vi "GLdrv_TRIG_COND_CH.vi"(0 "Connection ID":T2, 5 "COND":i32=1 min=0 max=1, 7 "CH":i32=1 min=1, 9 "Set":T1, 11 "error in (no error)":errorcluster, 13 "Query(f)":bool) -> (4 "Connection ID Out":T2, 10 "Set out":T1, 15 "error out":errorcluster)   [LabVIEW 2017, in "GL860_Driver.lvlib"]
doc: "トリガ SourceがAMPに設定されている場合、各アナログ入力CHのト\nリガのレベル値を設定します\nOFF：　トリガレベルを設定しません\nHI：　立上り（COMBがEDGE設定時）、以上（COMBがLEVEL設定時）\nLO： 立下り（COMBがEDGE設定時）、以下（COMBがLEVEL設定時）\nWIND,IN：　範囲内になったとき\nWIND,OUT：　範囲外になったとき\nTRIG:COND0:CH<CH値>:SET WIND,IN,<上限値>,<下限値>\n例)TRIG:COND0:CH2:SET HI,510C (スタートトリガのCH2をHIで\n510℃に設定します)\n例)TRIG:COND1:CH5:SET WIND,IN,+25.5MV,-12.4MV (ストップトリ\nガのCH5を範囲内で25.5mV～-12.4mVに設定します)"
uses:
  GL860_Driver.lvlib
  ConnectionID.ctl
  GLdrv_RW.ctl
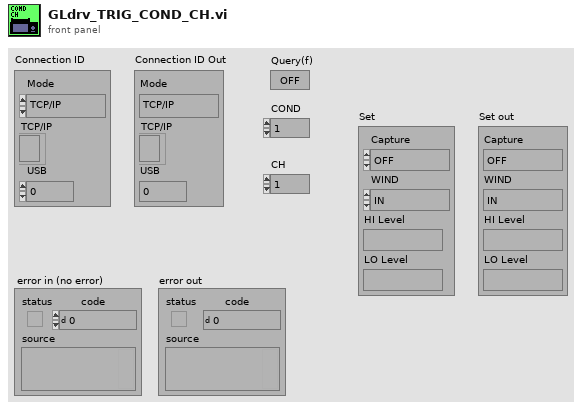
[diagram p1: front panel]
types:
  T1 = cluster{"Capture":enum16{"OFF", "HI", "LO", "WIND"}, "WIND":enum16{"IN", "OUT"}, "HI Level":string, "LO Level":string}
  T2 = typedef "ConnectionID.ctl" = cluster{"Mode":enum16{"TCP/IP", "USB"}, "TCP/IP":refnum<k5>, "USB":i32}
  T3 = typedef "GLdrv_RW.ctl" = enum16{"Auto", "Read", "Write", "Buffer"}
  T4 = cluster{"Capture":enum16{"OFF", "HI", "LO", "WIND"}, "WIND":enum16{"IN", "OUT"}, "data out":string, "data out":string}
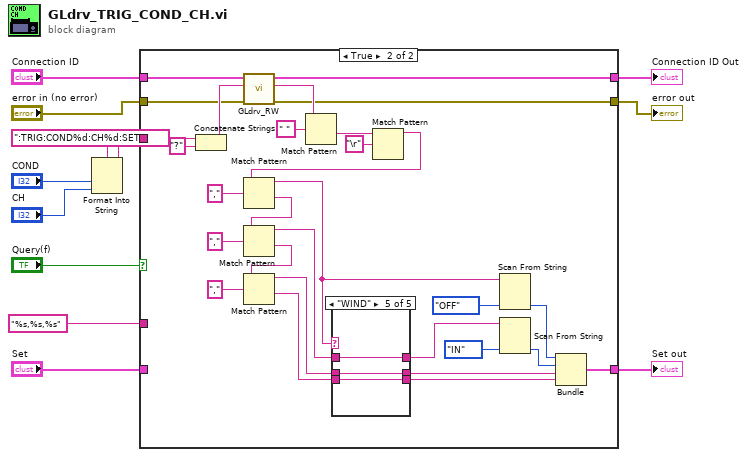
[diagram p0: block diagram]
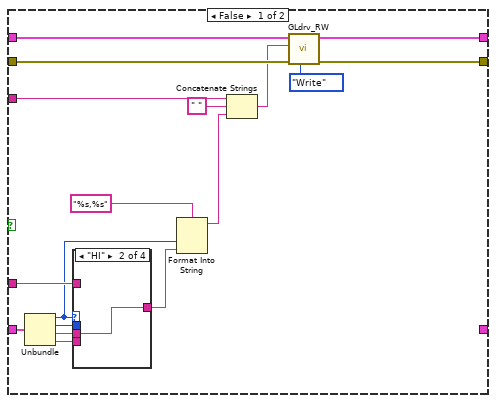
[diagram p2: hidden frame]
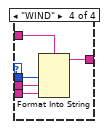
[diagram p5: hidden frame]
diagram:
  n1 = Format Into String(format string=":TRIG:COND%d:CH%d:SET" ("Command"), "COND", "CH") -> (resulting string=w7:string)  [unwired: 2 in, 1 out]
  n2 = case shown="TRUE" "Query(f)" {
    tunnel: w7 -> [w29 w62]
    tunnel: [w24 w55] -> w12
    tunnel: [w26 w59] -> w11
    tunnel: "Connection ID" -> [w27 w60]
    tunnel: "error in (no error)" -> [w25 w56]
    tunnel: [_ w43] -> w5
    tunnel: "Set" -> [w19 _]
    tunnel: "%s,%s,%s" ("format string") -> [w15 _]
    frame False {
      n3 = Unbundle(w19) -> ("Capture"=w14:enum16{"OFF", "HI", "LO", "WIND"}, "WIND"=w16:enum16{"IN", "OUT"}, "HI Level"=w18:string, "LO Level"=w20:string)
      n4 = case shown="\"HI\"" w14 {
        tunnel: w20 -> [_ _ w31 w34]
        tunnel: [_ w30 w31 w33] -> w17
        tunnel: w18 -> [_ w30 _ w36]
        tunnel: w16 -> [_ _ _ w35]
        tunnel: w15 -> [_ _ _ w32]
        frame "OFF" {
        }
        frame "HI" {
        }
        frame "LO" {
        }
        frame "WIND" {
          n5 = Format Into String(format string=w32, w35, w36, w34) -> (resulting string=w33:string)  [unwired: 2 in, 1 out]
        }
      }
      n6 = Format Into String(format string="%s,%s" ("Param"), w14, w17) -> (resulting string=w21:string)  [unwired: 2 in, 1 out]
      n7 = Concatenate Strings(w29, " " ("string"), w21) -> (w23:string)
      n8 = call "GLdrv_RW.vi"("Mode(read)"=GLdrv_RW."Write", "error in (no error)"=w25, "data in"=w23, "Connection ID"=w27) -> ("error out"=w24:errorcluster, "Connection ID Out"=w26:T2)  [unwired: 3 in, 3 out]
    }
    frame True {
      n9 = Concatenate Strings(w62, "?" ("string")) -> (w58:string)
      n10 = call "GLdrv_RW.vi"("error in (no error)"=w56, "data in"=w58, "Connection ID"=w60) -> ("error out"=w55:errorcluster, "data out"=w57:string, "Connection ID Out"=w59:T2)  [unwired: 4 in, 2 out]
      n11 = Match Pattern(string=w57, regular expression=" " ("search string/char (-)")) -> (after substring=w63:string)  [unwired: 4 out]
      n12 = Match Pattern(string=w63, regular expression="\r") -> (before substring=w49:string)  [unwired: 4 out]
      n13 = Match Pattern(string=w49, regular expression=",") -> (before substring=w46:string, after substring=w51:string)  [unwired: 3 out]
      n14 = Match Pattern(string=w51, regular expression=",") -> (before substring=w48:string, after substring=w50:string)  [unwired: 3 out]
      n15 = Match Pattern(string=w50, regular expression=",") -> (before substring=w47:string, after substring=w39:string)  [unwired: 3 out]
      n16 = case shown="\"WIND\"" w46 {
        tunnel: w48 -> [_ _ w66 w67 w70]
        tunnel: w47 -> [_ _ _ _ w69]
        tunnel: w39 -> [_ _ _ _ w68]
        tunnel: [_ _ _ _ w70] -> w40
        tunnel: [_ _ w66 _ w69] -> w38
        tunnel: [_ _ _ w67 w68] -> w37
        frame Default {
        }
        frame "OFF" {
        }
        frame "HI" {
        }
        frame "LO" {
        }
        frame "WIND" {
        }
      }
      n17 = Scan From String(input string=w46, default 1=enum16{"OFF", "HI", "LO", "WIND"}."OFF" ("Capture")) -> (output 1=w45:enum16{"OFF", "HI", "LO", "WIND"})  [unwired: 3 in, 3 out]
      n18 = Scan From String(input string=w40, default 1=enum16{"IN", "OUT"}."IN" ("WIND")) -> (output 1=w41:enum16{"IN", "OUT"})  [unwired: 3 in, 3 out]
      n19 = Bundle("Capture"=w45, "WIND"=w41, "data out"=w38, "data out"=w37) -> (w43:T4)  [unwired: 1 out]
    }
  }
  "Connection ID Out" <- w11
  "error out" <- w12
  "Set out" <- w5
